vi "zad2.vi"() -> ()   [LabVIEW 2017]
panel:
  out "Waveform Graph":dynamicdata(graph)
  in  "Amplituda szumu":dbl
  in  "Czestotliwosc":dbl
  in  "Amplituda":dbl
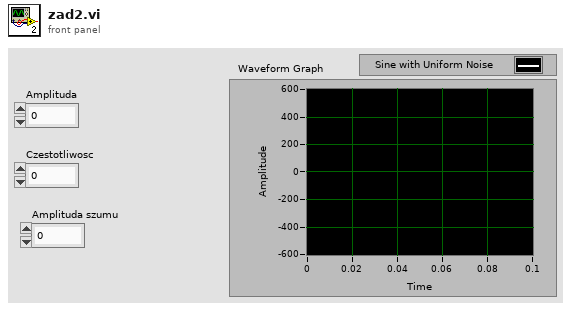
[diagram p1: front panel]
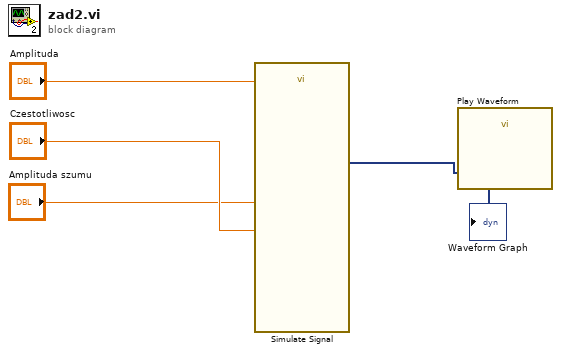
[diagram p0: block diagram]
diagram:
  n1 = call "Simulate Signal"("Frequency"="Czestotliwosc", "Amplitude"="Amplituda", "Noise amplitude"="Amplituda szumu") -> ("Sine with Uniform Noise"=w1:dynamicdata)  [unwired: 11 in, 1 out]
  "Waveform Graph" <- w1
  n2 = call "Play Waveform"("Data"=w1) -> ()  [unwired: 18 in, 1 out]
